vi "Is Valid Item.vi"(8 "error in (no error)":errorcluster, 10 "Item ID":string, 11 "VI in":refnum<class "VI.lvclass">) -> (0 "error out":errorcluster, 1 "Is Valid?":bool, 2 "Is Item?":bool, 3 "VI out":refnum<class "VI.lvclass">)   [LabVIEW 2020, in "VI Properties Editor.lvlib" / "VI.lvclass"]
doc: "Checks if <B>VI in</B> is identified by <B>Item ID</B> and checks if it is a valid item, meaning one that is able to be edited in the application."
uses:
  VI.lvclass
  C:/Users/acasalen/Documents/LabVIEW Data/Projects/VI-Properties-Editor/source/Classes/Item/Item.lvclass
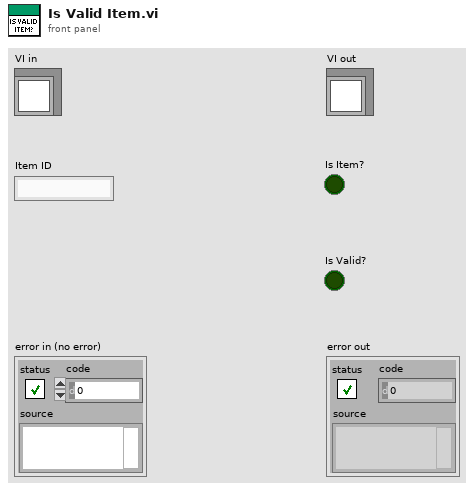
[diagram p1: front panel]
types:
  T1 = enum32{"invalid VI type", "Standard VI", "Control VI", "Global VI", "Polymorphic VI", "Configuration VI", "SubSystem", "Facade VI", "Method VI", "Statechart Diagram VI"}[]
  T2 = enum32{"invalid VI type", "Standard VI", "Control VI", "Global VI", "Polymorphic VI", "Configuration VI", "SubSystem", "Facade VI", "Method VI", "Statechart Diagram VI"}
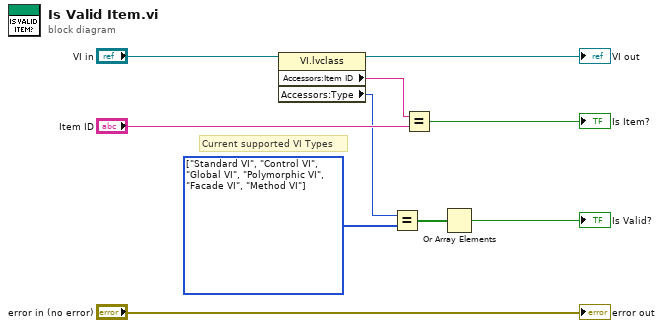
[diagram p0: block diagram]
diagram:
  w3 = T1 [enum."Standard VI", enum."Control VI", enum."Global VI", enum."Polymorphic VI", enum."Facade VI", enum."Method VI"] items=["invalid VI type", "Standard VI", "Control VI", "Global VI", "Polymorphic VI", "Configuration VI", "SubSystem", "Facade VI", "Method VI", "Statechart Diagram VI"]
  # "Current supported VI Types"
  n1 = property class="VI.lvclass"(reference="VI in") -> (reference out=→"VI out":refnum<class "VI.lvclass">, "Accessors:Item ID"=w8:string, "Accessors:Type"=w4:T2)  [unwired: 1 in, 1 out]
  n2 = Equal?(x=w4, y=w3) -> (x = y?=w2:bool[])
  n3 = Equal?(x=w8, y="Item ID") -> (x = y?=→"Is Item?":bool)
  n4 = Or Array Elements(Boolean array=w2) -> (logical OR=→"Is Valid?":bool)
  "error out" <- "error in (no error)"
